vi "ExpOpen.vi"(6 "Show Labview Expose Logs":bool, 7 "Timeout (ms)":i32=10000, 8 "error in (no error)":errorcluster, 9 "Do Expose Logging":bool, 10 "Requires Matlab Enviroment":bool, 11 "Experiment file path (or root calling vi)":path) -> (0 "error out":errorcluster, 2 "Experiment Info":T1={"ExposeInfo"={"CSCom"=refnum, "URL"="", "Events Category"="", "ID"="", "SRefID"=""}, "ExpID"="[noexp]", "ExperimentFilename"="", "Caller Keep Alive"=refnum}, 3 "ExpID":string)   [LabVIEW 2017]
uses:
  ExperimentInfo.ctl
  Expose/Labview/Core/ExposeInfo.ctl
  C:/Code/CMCryoSysCode/Expose/COM/CSCom/CSCom/bin/Release/CSCom.dll
  Expose/COM/CSCom/CSCom/bin/Release/CSCom.dll
  Expose/Labview/Core/ExposeGlobals.vi
  ExpGlobals.vi
panel:
  out "Experiment File":string
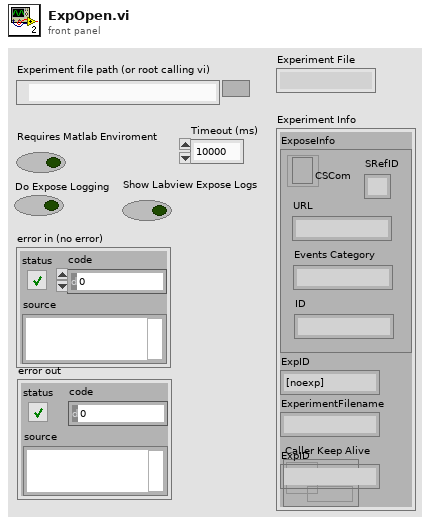
[diagram p1: front panel]
types:
  T1 = typedef "ExperimentInfo.ctl" = cluster{"ExposeInfo":T2, "ExpID":string, "ExperimentFilename":string, "Caller Keep Alive":refnum<data-value>}
  T2 = typedef "ExposeInfo.ctl" = cluster{"CSCom":refnum<k24>, "URL":string, "Events Category":string, "ID":string, "SRefID":string}
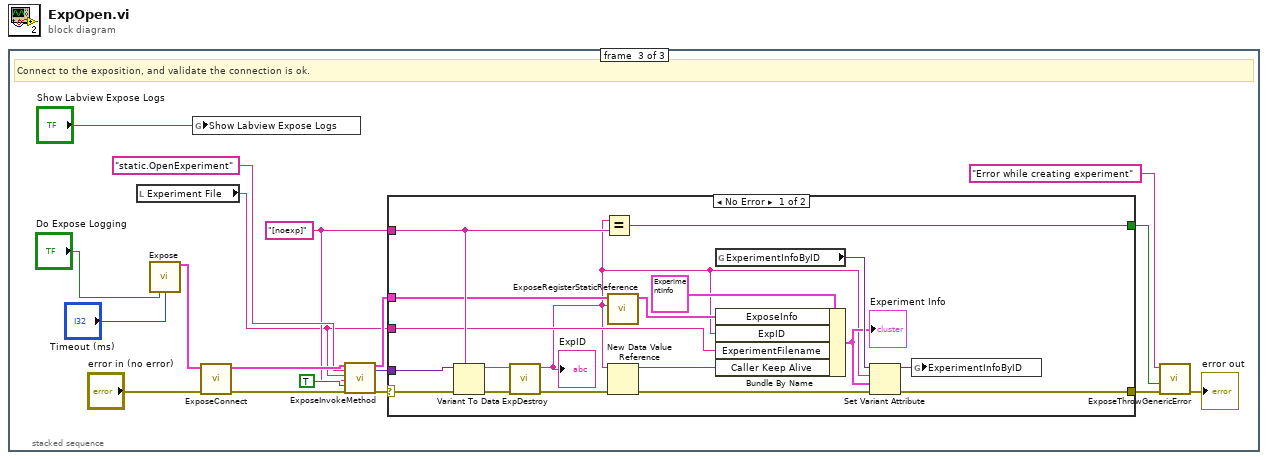
[diagram p0: block diagram]
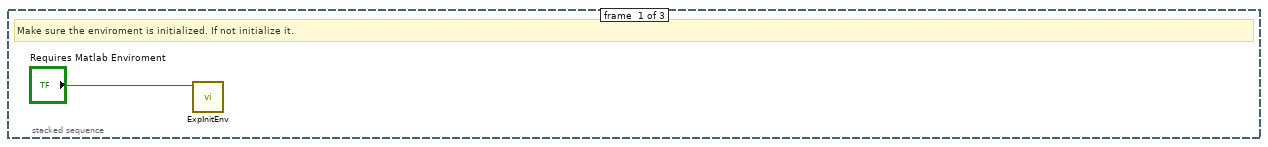
[diagram p2: hidden frame]
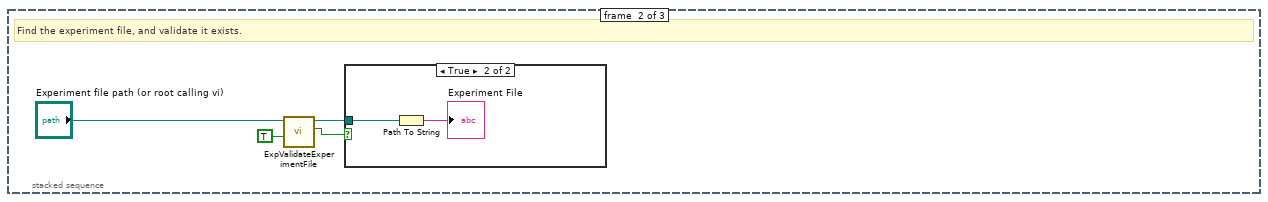
[diagram p3: hidden frame]
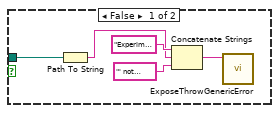
[diagram p4: hidden frame]
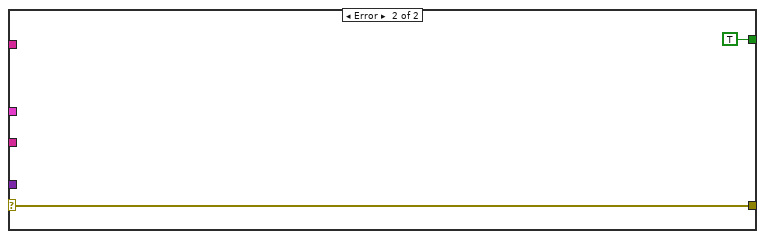
[diagram p5: hidden frame]
diagram:
  n1 = stacked-sequence {
    frame #0 {
      # "Make sure the enviroment is initialized. If not initialize it."
      n2 = call "ExpInitEnv.vi"("Requires Matlab Enviroment"="Requires Matlab Enviroment") -> ()  [unwired: 10 in, 1 out]
    }
    frame #1 {
      # "Find the experiment file, and validate it exists."
      n3 = call "ExpValidateExperimentFile.vi"("AsSubCaller"=TRUE, "Experiment file path (or root calling vi)"="Experiment file path (or root calling vi)") -> ("Found?"=w5:bool, "Experiment File path"=w3:path)  [unwired: 8 in]
      n4 = case shown="True" w5 {
        tunnel: w3 -> [w7 w12]
        frame False {
          n5 = Path To String(path=w7) -> (string=w6:string)
          n6 = Concatenate Strings("Experiment file '" ("string"), w6, "' not found. Please provide an experiment file path." ("string")) -> (w8:string)
          n7 = call "ExposeThrowGenericError.vi"("TheError"=w8) -> ()  [unwired: 10 in, 1 out]
        }
        frame True {
          n8 = Path To String(path=w12) -> (string=→"Experiment File":string)
        }
      }
    }
    frame #2 {
      w24 = "[noexp]" ("Text")
      # "Connect to the exposition, and validate the connection is ok."
      n9 = local read "Experiment File"() -> (w21:string)
      n10 = call "Expose.vi"("DoLogging"="Do Expose Logging", "Timeout (ms)"="Timeout (ms)") -> ("Expose"=w29:T2)  [unwired: 13 in]
      n11 = global write "ExposeGlobals.vi" "Show Labview Expose Logs"("Show Labview Expose Logs") -> ()
      n12 = call "ExposeConnect.vi"("error in (no error)"="error in (no error)", "Expose Info"=w29) -> ("error out"=w20:errorcluster, "Expose Info out"=w28:T2)  [unwired: 8 in]
      n13 = call "ExposeInvokeMethod.vi"("Expose Info in"=w28, "Method Name"="static.OpenExperiment" ("Text"), "Argument(s)"=w21, "Rsp. Type (or value to update)"=w24, "Require Response"=TRUE, "error in (no error)"=w20) -> ("Expose out"=w22:T2, "Response"=w25:variant, "error out"=w19:errorcluster)  [unwired: 11 in]
      n14 = case shown="No Error" w19 {
        selector: w19 -> [w38 w49]
        tunnel: w25 -> [w48 _]
        tunnel: w24 -> [w47 _]
        tunnel: [w46 TRUE] -> w23
        tunnel: w22 -> [w34 _]
        tunnel: w21 -> [w44 _]
        tunnel: [w35 w49] -> w13
        frame No Error {
          n15 = Variant To Data(error in=w38, type=w47, Variant=w48) -> (data=w32:string, error out=w39:errorcluster)
          n16 = call "ExpDestroy.vi"("error in"=w39, "ExpID"=w32) -> ("error out"=w37:errorcluster, "ExpID out"=w31:string)  [unwired: 8 in]
          "ExpID" <- w31
          n17 = Equal?(x=w31, y=w47) -> (x = y?=w46:bool)
          n18 = call "ExposeRegisterStaticReference.vi"("Static refrence ID"=w31, "Expose Info"=w34) -> ("Expose Info out"=w33:T2)  [unwired: 9 in]
          n19 = New Data Value Reference(data value=w31, error in=w37) -> (data value reference=w40:refnum<data-value>, error out=w36:errorcluster)
          n20 = global read "ExpGlobals.vi" "ExperimentInfoByID"() -> (w43:variant)
          n21 = Bundle By Name(cluster=T1 {"ExposeInfo"={"CSCom"=refnum, "URL"="", "Events Category"="", "ID"="", "SRefID"=""}, "ExpID"="[noexp]", "ExperimentFilename"="", "Caller Keep Alive"=refnum} ("ExperimentInfo"), "ExposeInfo"=w33, "ExpID"=w31, "ExperimentFilename"=w44, "Caller Keep Alive"=w40) -> (w41:T1)
          "Experiment Info" <- w41
          n22 = Set Variant Attribute(Variant=w43, name=w31, value=w41, error in=w36) -> (Variant out=w42:variant, error out=w35:errorcluster)  [unwired: 1 out]
          n23 = global write "ExpGlobals.vi" "ExperimentInfoByID"(w42) -> ()
        }
        frame Error {
        }
      }
      n24 = call "ExposeThrowGenericError.vi"("error in (no error)"=w13, "Invoke?"=w23, "TheError"="Error while creating experiment") -> ("error out"=→"error out":errorcluster)  [unwired: 8 in]
    }
  }
